vi "SmartMove-Communication.vi"(5 "Option":enum16{"nothing", "get", "set", "send raw"}(ring), 6 "error in":errorcluster, 7 "Value":string, 8 "Parameter":string, 9 "VISA resource 2":refnum<visa-resource-name>) -> (0 "error out":errorcluster, 2 "read value/raw":string, 3 "VISA resource":refnum<visa-resource-name>)   [LabVIEW 8.6]
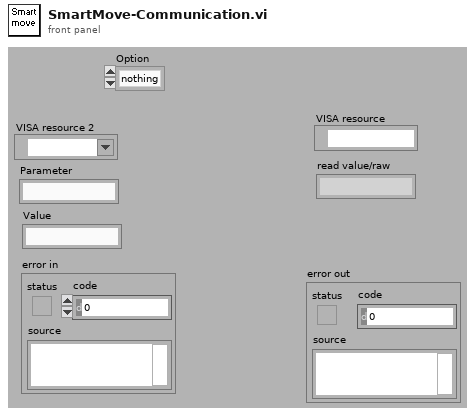
[diagram p1: front panel]
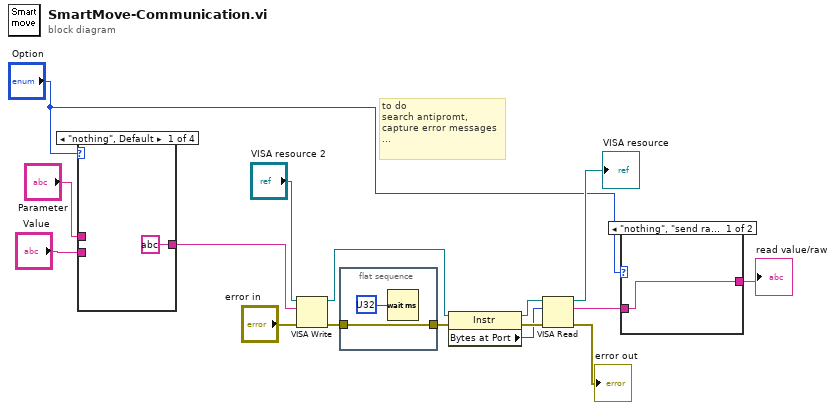
[diagram p0: block diagram]
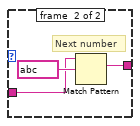
[diagram p2: hidden frame]
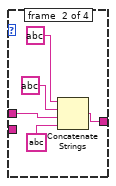
[diagram p3: hidden frame]
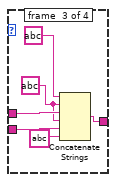
[diagram p4: hidden frame]
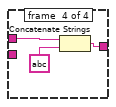
[diagram p5: hidden frame]
diagram:
  # "to do \nsearch antipromt,\ncapture error messages\n..."
  n1 = case shown="\"nothing\", Default" "Option" {
    tunnel: "Value" -> [_ _ w28 _]
    tunnel: [string ? w21 w26 w30] -> w8
    tunnel: "Parameter" -> [_ w20 w25 w29]
    frame #0 {
    }
    frame #1 {
      n2 = Concatenate Strings(string ?, string ?, w20, string ?) -> (w21:string)
    }
    frame #2 {
      w23 = string ?
      n3 = Concatenate Strings(string ?, w23, w25, w23, w28, string ?) -> (w26:string)
    }
    frame #3 {
      n4 = Concatenate Strings(w29, string ?) -> (w30:string)
    }
  }
  n5 = VISA Write(VISA resource name="VISA resource 2", write buffer=w8, error in (no error)="error in") -> (VISA resource name out=w4:refnum<visa-resource-name>, error out=w3:errorcluster)  [unwired: 1 out]
  n6 = flat-sequence {
    tunnel: w3 -> [w32]
    tunnel: [w32] -> w5
    frame #0 {
      n7 = Wait (ms)(milliseconds to wait=u32 ?) -> ()  [unwired: 1 out]
    }
  }
  n8 = property class="Instr"(reference=w4, error in=w5) -> (reference out=w6:refnum<visa-resource-name>, error out=w15:errorcluster, "Bytes at Port"=w7:u32)
  n9 = VISA Read(VISA resource name=w6, byte count=w7, error in (no error)=w15) -> (VISA resource name out=→"VISA resource":refnum<visa-resource-name>, read buffer=w12:string, error out=→"error out":errorcluster)  [unwired: 1 out]
  n10 = case shown="\"nothing\", \"send raw\"" "Option" {
    tunnel: [w34 w37] -> w16
    tunnel: w12 -> [w34 w35]
    frame #0 {
    }
    frame #1 {
      # "Next number"
      n11 = Match Pattern(string=w35, regular expression=string ?) -> (match substring=w37:string)  [unwired: 4 out]
    }
  }
  "read value/raw" <- w16
